vi "drawIntensityGraph.vi"(6 "color(black)":u32(colorbox), 9 "Combo Box":string(combo), 10 "Coords":T1, 11 "Left Graph 2":refnum<vi>) -> (2 "y":i32, 3 "x":i32)   [LabVIEW 2016]
uses:
  <vilib>/Utility/miscctls.llb/LVPoint32TypeDef.ctl
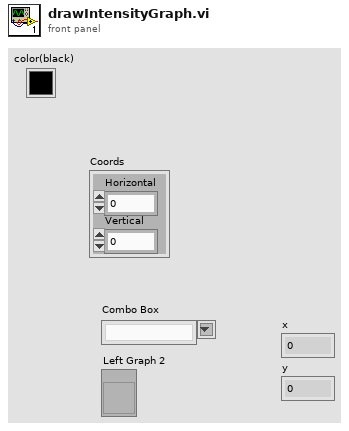
[diagram p1: front panel]
types:
  T1 = typedef "LVPoint32TypeDef.ctl" = cluster{"Horizontal":i32, "Vertical":i32}
  T2 = cluster{"Width":u16, "Style":enum32{"Solid", "Dash", "Dot", "DashDot", "DashDotDot"}}
  T3 = typedef "LVRectTypeDef.ctl" = cluster{"Left":i16, "Top":i16, "Right":i16, "Bottom":i16}
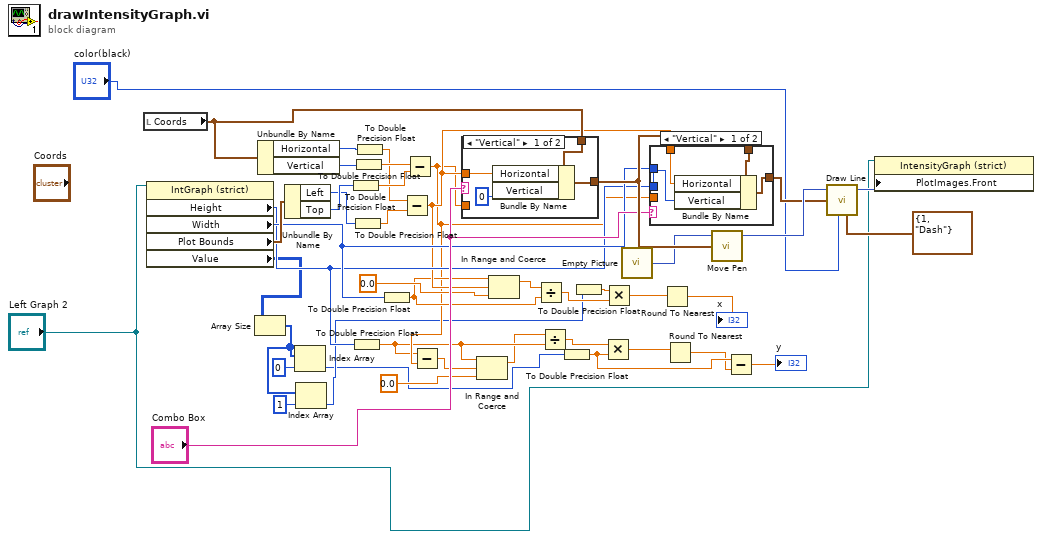
[diagram p0: block diagram]
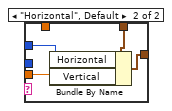
[diagram p2: hidden frame]
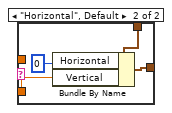
[diagram p3: hidden frame]
diagram:
  n1 = local read "Coords"() -> (w39:T1)
  n2 = property class="IntGraph (strict)"(reference="Left Graph 2") -> ("Height"=w27:u32, "Width"=w28:u32, "Plot Bounds"=w29:T3, "Value"=w17:i32[][])  [unwired: 1 in, 2 out]
  n3 = Array Size(array=w17) -> (size(s)=w14:i32[])
  n4 = Unbundle By Name(w39) -> ("Horizontal"=w33:i32, "Vertical"=w41:i32)
  n5 = Unbundle By Name(w29) -> ("Left"=w34:i16, "Top"=w40:i16)
  n6 = Index Array(array=w14, index=0) -> (element=w2:i32)
  n7 = Index Array(array=w14, index=1) -> (element=w3:i32)
  n8 = To Double Precision Float(number=w40) -> (double precision float=w37:dbl)
  n9 = To Double Precision Float(number=w27) -> (double precision float=w19:dbl)
  n10 = To Double Precision Float(number=w34) -> (double precision float=w31:dbl)
  n11 = To Double Precision Float(number=w41) -> (double precision float=w38:dbl)
  n12 = To Double Precision Float(number=w33) -> (double precision float=w30:dbl)
  n13 = To Double Precision Float(number=w28) -> (double precision float=w24:dbl)
  n14 = Subtract(x=w30, y=w31) -> (x-y=w26:dbl)
  n15 = Subtract(x=w38, y=w37) -> (x-y=w22:dbl)
  n16 = Subtract(x=w19, y=w22) -> (x-y=w21:dbl)
  n17 = case shown="\"Vertical\"" "Combo Box" {
    tunnel: [w48 w52] -> w43
    tunnel: w39 -> [w49 w51]
    tunnel: w22 -> [_ w50]
    tunnel: w26 -> [w46 _]
    frame "Vertical" {
      n18 = Bundle By Name(cluster=w49, "Horizontal"=w46, "Vertical"=0) -> (w48:T1)
    }
    frame "Horizontal", Default {
      n19 = Bundle By Name(cluster=w51, "Horizontal"=0, "Vertical"=w50) -> (w52:T1)
    }
  }
  n20 = In Range and Coerce(upper limit=w19, x=w21, lower limit=0.0) -> (coerced(x)=w18:dbl)  [unwired: 1 out]
  n21 = In Range and Coerce(upper limit=w24, x=w26, lower limit=0.0) -> (coerced(x)=w23:dbl)  [unwired: 1 out]
  n22 = Divide(x=w23, y=w24) -> (x/y=w15:dbl)
  n23 = Divide(x=w18, y=w19) -> (x/y=w12:dbl)
  n24 = To Double Precision Float(number=w2) -> (double precision float=w5:dbl)
  n25 = To Double Precision Float(number=w3) -> (double precision float=w11:dbl)
  n26 = Multiply(x=w12, y=w5) -> (x*y=w9:dbl)
  n27 = Multiply(x=w11, y=w15) -> (x*y=w10:dbl)
  n28 = call "Empty Picture"() -> ("empty picture"=w35:picture)
  n29 = case shown="\"Vertical\"" "Combo Box" {
    tunnel: w43 -> [w57 w61]
    tunnel: [w56 w60] -> w42
    tunnel: w28 -> [_ w59]
    tunnel: w22 -> [_ w58]
    tunnel: w26 -> [w55 _]
    tunnel: w27 -> [w54 _]
    frame "Vertical" {
      n30 = Bundle By Name(cluster=w57, "Horizontal"=w55, "Vertical"=w54) -> (w56:T1)
    }
    frame "Horizontal", Default {
      n31 = Bundle By Name(cluster=w61, "Horizontal"=w59, "Vertical"=w58) -> (w60:T1)
    }
  }
  n32 = Round To Nearest(number=w10) -> (nearest integer value=→"x":dbl)
  n33 = Round To Nearest(number=w9) -> (nearest integer value=w4:dbl)
  n34 = call <vilib>:"Move Pen.vi"("new position"=w43, "picture"=w35) -> ("new picture"=w45:picture)  [unwired: 3 in]
  n35 = Subtract(x=w5, y=w4) -> (x-y=→"y":dbl)
  n36 = call <vilib>:"Draw Line.vi"("picture"=w45, "end point"=w42, "color(black)"="color(black)", "pen"=T2 {"Width"=1, "Style"=enum."Dash"}) -> ("new picture"=w36:picture)  [unwired: 5 in]
  n37 = property on="Property Node" class="IntensityGraph (strict)"(reference="Left Graph 2", "PlotImages.Front"=w36) -> ()  [unwired: 1 in, 2 out]
